vi "Read.vi"(0 "reference in":refnum<class "Barcode_Reader_Dialog.lvclass">, 5 "error in (no error)":errorcluster) -> (14 "reference in":refnum<class "Barcode_Reader_Dialog.lvclass">, 16 "Serial":string, 17 "read Ok":bool, 19 "error out":errorcluster)   [LabVIEW 2022 SP3, in "Barcode_Reader_Dialog.lvlib" / "Barcode_Reader_Dialog.lvclass"]
uses:
  Barcode_Reader_Dialog.lvclass
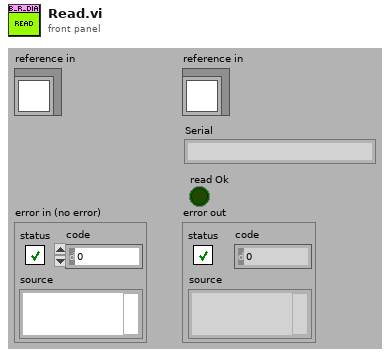
[diagram p1: front panel]
types:
  T1 = typedef "Barcode_Reader_Dialog.lvlib/Barcode_Reader_Dialog.lvclass/ObjectAttributes.ctl" = cluster{"Config":T2, "Serial":string}
  T2 = typedef "Barcode_Reader_Dialog.lvlib/Barcode_Reader_Dialog.lvclass/Config.ctl" = cluster{"default":string}
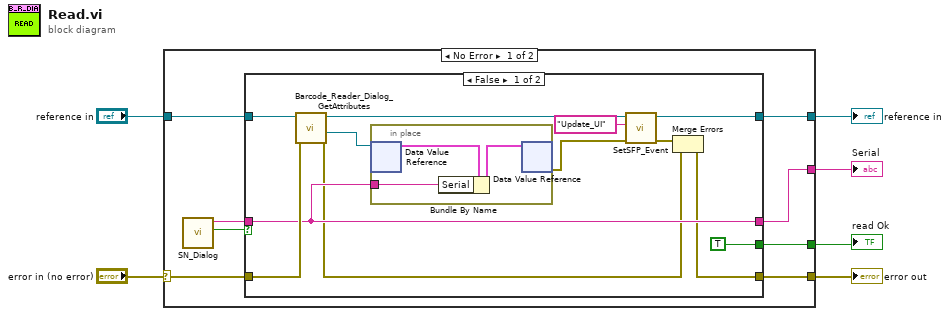
[diagram p0: block diagram]
diagram:
  n1 = case shown="No Error" "error in (no error)" {
    selector: "error in (no error)" -> [w14 w33]
    tunnel: [w13 w33] -> w5
    tunnel: [w11 w32] -> w3
    tunnel: "reference in" -> [w12 w32]
    tunnel: [w8 _] -> w2
    tunnel: [w7 _] -> w1
    frame No Error {
      n2 = call "SN_Dialog.vi"() -> ("Cancelled"=w10:bool, "UserName"=w9:string)  [unwired: 10 in]
      n3 = case shown="False" w10 {
        tunnel: w14 -> [w26 w31]
        tunnel: [w15 w31] -> w13
        tunnel: w12 -> [w25 w30]
        tunnel: [w20 w30] -> w11
        tunnel: w9 -> [w23 _]
        tunnel: [w23 _] -> w8
        tunnel: [TRUE _] -> w7
        frame False {
          n4 = call "Barcode_Reader_Dialog_GetAttributes.vi"("error in (no error)"=w26, "reference in"=w25) -> ("error out"=w16:errorcluster, "DataRef"=w24:refnum<data-value>, "reference out"=w21:refnum<class "Barcode_Reader_Dialog.lvclass">)  [unwired: 6 in, 1 out]
          n5 = in-place {
            in-place-border: w23 -> [w27]
            n6 = in-place-dvr #1(w24) -> (w29:T1)  [unwired: 1 out]
            n7 = Bundle By Name(cluster=w29, "Serial"=w27) -> (w28:T1)
            n8 = in-place-dvr #1(w28) -> (w19:errorcluster)  [unwired: 1 out]
          }
          n9 = call-dynamic "SetSFP_Event.vi"("error in (no error)"=w19, "msg"="Update_UI", "reference in"=w21) -> ("error out"=w17:errorcluster, "reference out"=w20:refnum<class "Barcode_Reader_Dialog.lvclass">)  [unwired: 7 in]
          n10 = Merge Errors(w17, w16) -> (w15:errorcluster)
        }
        frame True {
        }
      }
    }
    frame Error {
    }
  }
  "error out" <- w5
  "reference in" <- w3
  "Serial" <- w2
  "read Ok" <- w1
